vi "action.vi"(8 "error in":errorcluster, 9 "status":T1=enum."Validate", 10 "Input":string, 11 "Users indicate":T3) -> (0 "error out":errorcluster, 1 "Message":T2, 2 "Result":string, 3 "Users indicate  2":T3)   [LabVIEW 2015]
doc: "Generate proper action for withdraw, deposit maoney and user validation."
uses:
  controls/users ind.ctl
  controls/user.ctl
  controls/message.ctl
  controls/nextstate.ctl
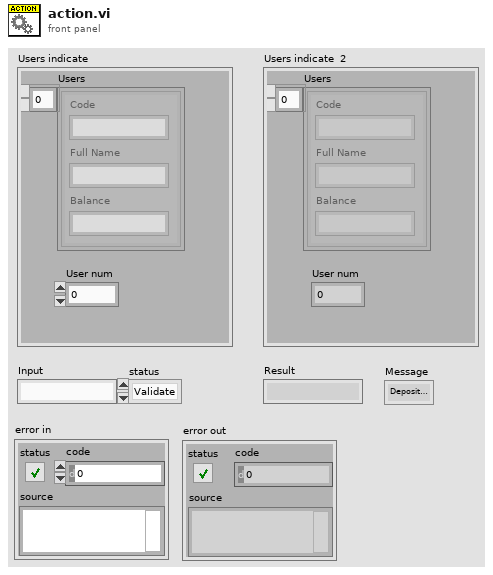
[diagram p1: front panel]
types:
  T1 = typedef "nextstate.ctl" = enum16{"Fast Cash", "Withdraw", "Deposit", "Validate"}
  T2 = typedef "message.ctl" = enum16{"Deposit Complete", "Welcome", "Menu", "Verification Failed", "Session Terminate", "Deposit", "Withdrawal", "Withdrawal Complete", "Withdrawal Failed", "Balance Inq"}
  T3 = typedef "users ind.ctl" = cluster{"Users":T4[], "User num":i32}
  T4 = typedef "user.ctl" = cluster{"Code":string, "Full Name":string, "Balance":string}
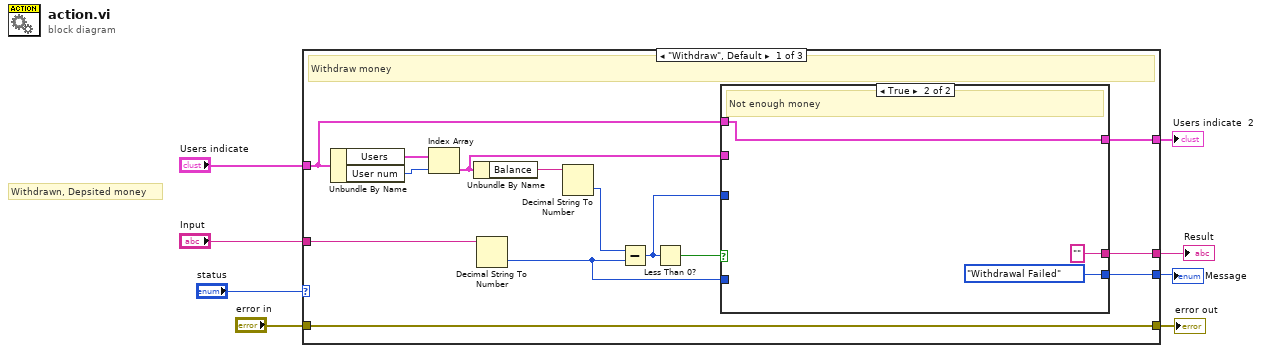
[diagram p0: block diagram]
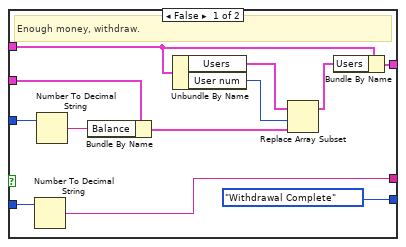
[diagram p2: hidden frame]
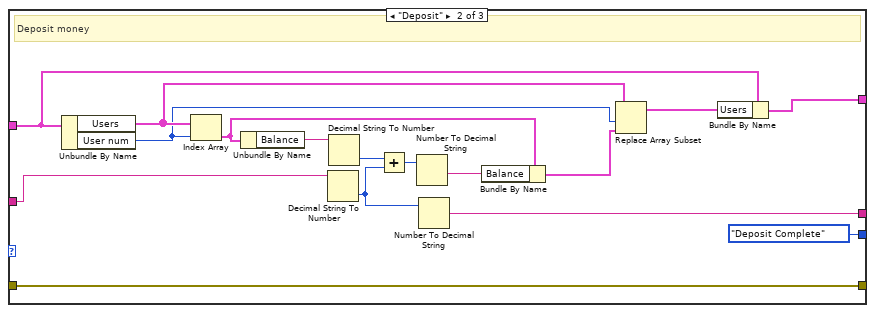
[diagram p3: hidden frame]
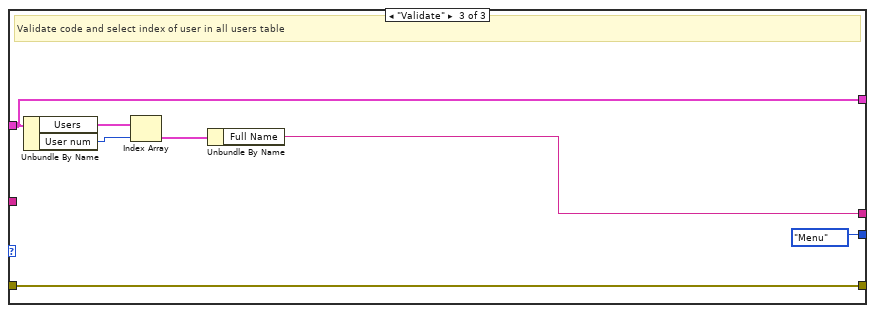
[diagram p4: hidden frame]
diagram:
  # "Withdrawn, Depsited money"
  n1 = case shown="\"Withdraw\", Default" "status" {
    tunnel: "Users indicate" -> [w15 w49 w55]
    tunnel: [w11 w38 w57] -> w5
    tunnel: "Input" -> [w19 w52 _]
    tunnel: [w16 message."Deposit Complete" ("Message") message."Menu" ("Message")] -> w8
    tunnel: [w12 w45 w55] -> w7
    tunnel: "error in" -> [w10 w40 w54]
    tunnel: [w10 w40 w54] -> w1
    frame "Withdraw", Default {
      # "Withdraw money"
      n2 = Unbundle By Name(w15) -> ("Users"=w22:T4[], "User num"=w21:i32)
      n3 = Index Array(array=w22, index=w21) -> (element=w14:T4)
      n4 = Unbundle By Name(w14) -> ("Balance"=w20:string)
      n5 = Decimal String To Number(string=w19) -> (number=w9:i32)  [unwired: 2 in, 1 out]
      n6 = Decimal String To Number(string=w20) -> (number=w18:i32)  [unwired: 2 in, 1 out]
      n7 = Subtract(x=w18, y=w9) -> (x-y=w13:i32)
      n8 = Less Than 0?(x=w13) -> (x < 0?=w17:bool)
      n9 = case shown="True" w17 {
        tunnel: [message."Withdrawal Complete" ("Message") message."Withdrawal Failed" ("Message")] -> w16
        tunnel: w15 -> [w33 w36]
        tunnel: w14 -> [w28 _]
        tunnel: w13 -> [w32 _]
        tunnel: [w25 w36] -> w12
        tunnel: [w23 ""] -> w11
        tunnel: w9 -> [w24 _]
        frame False {
          # "Enough money, withdraw."
          n10 = Number To Decimal String(number=w24) -> (decimal integer string=w23:string)  [unwired: 1 in]
          n11 = Number To Decimal String(number=w32) -> (decimal integer string=w27:string)  [unwired: 1 in]
          n12 = Bundle By Name(cluster=w28, "Balance"=w27) -> (w26:T4)
          n13 = Unbundle By Name(w33) -> ("Users"=w30:T4[], "User num"=w31:i32)
          n14 = Replace Array Subset(array=w30, new element=w26, index=w31) -> (w29:T4[])
          n15 = Bundle By Name(cluster=w33, "Users"=w29) -> (w25:T3)
        }
        frame True {
          # "Not enough money"
        }
      }
    }
    frame "Deposit" {
      # "Deposit money"
      n16 = Unbundle By Name(w49) -> ("Users"=w48:T4[], "User num"=w47:i32)
      n17 = Index Array(array=w48, index=w47) -> (element=w44:T4)
      n18 = Unbundle By Name(w44) -> ("Balance"=w53:string)
      n19 = Decimal String To Number(string=w52) -> (number=w39:i32)  [unwired: 2 in, 1 out]
      n20 = Decimal String To Number(string=w53) -> (number=w51:i32)  [unwired: 2 in, 1 out]
      n21 = Add(x=w51, y=w39) -> (x+y=w50:i32)
      n22 = Number To Decimal String(number=w50) -> (decimal integer string=w42:string)  [unwired: 1 in]
      n23 = Number To Decimal String(number=w39) -> (decimal integer string=w38:string)  [unwired: 1 in]
      n24 = Bundle By Name(cluster=w44, "Balance"=w42) -> (w43:T4)
      n25 = Replace Array Subset(array=w48, new element=w43, index=w47) -> (w46:T4[])
      n26 = Bundle By Name(cluster=w49, "Users"=w46) -> (w45:T3)
    }
    frame "Validate" {
      # "Validate code and select index of user in all users table"
      n27 = Unbundle By Name(w55) -> ("Users"=w60:T4[], "User num"=w59:i32)
      n28 = Index Array(array=w60, index=w59) -> (element=w58:T4)
      n29 = Unbundle By Name(w58) -> ("Full Name"=w57:string)
    }
  }
  "Result" <- w5
  "Users indicate  2" <- w7
  "Message" <- w8
  "error out" <- w1
